vi "oa_Attach Pulse Position Info.vi"(0 "speed profile signal input":waveform(dbl)={"t0"=timestamp(0 s since 1904-01-01), "dt"=0.0, "Y"=[]}, 5 "pulse/revolution (1)":i32, 7 "Rotation direction":u16(ring) caption="rotation direction  (CCW)" items=["CCW", "CW"], 9 "speed profile input":T1 {"speed [RPM]" format="%.2f"; "time [s]" format="%.2f"}, 11 "error in (no error)":errorcluster) -> (4 "speed profile":waveform(dbl), 15 "error out":errorcluster)   [LabVIEW 2017, in "SoundVib_TachProcess.lvlib"]
uses:
  <vilib>/addons/Sound and Vibration/Order Analysis/Tach Process/SoundVib_TachProcess.lvlib
  <vilib>/addons/Sound and Vibration/Order Analysis/Tach Process/SubVIs/speed profile.ctl
panel:
  in  "Waveform":waveform(dbl)={"t0"=timestamp(0 s since 1904-01-01), "dt"=0.0, "Y"=[], "attributes"=variant("NI_OA_Pulse_Per_Rev"=variant(i32 1), "NI_OA_Rotation_Direction"=variant(u16 0), "NI_OA_Speed_Profile"=variant(cluster{"time [s]":dbl[], "speed [RPM]":dbl[]} {"time [s]"=[], "speed [RPM]"=[]}))}
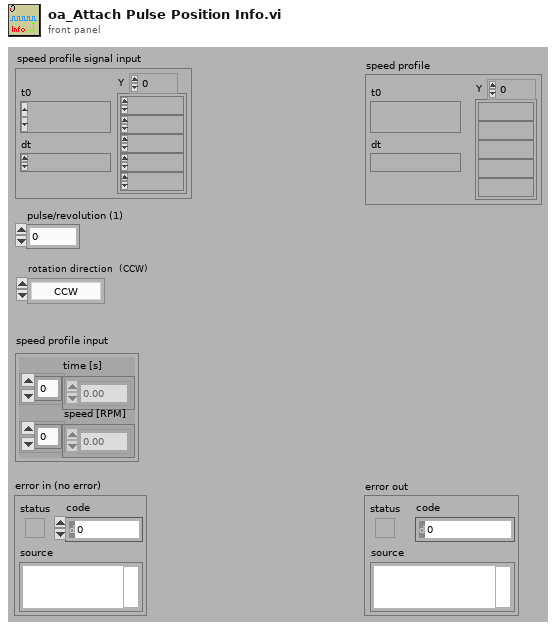
[diagram p1: front panel]
types:
  T1 = typedef "SoundVib_TachProcess.lvlib/speed profile.ctl" = cluster{"time [s]":dbl[], "speed [RPM]":dbl[]}
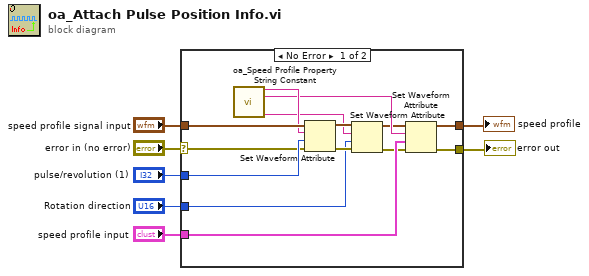
[diagram p0: block diagram]
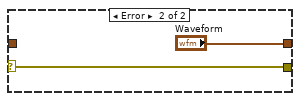
[diagram p2: hidden frame]
diagram:
  n1 = case shown="No Error" "error in (no error)" {
    selector: "error in (no error)" -> [w16 w23]
    tunnel: "speed profile signal input" -> [w21 _]
    tunnel: "pulse/revolution (1)" -> [w20 _]
    tunnel: [w19 "Waveform"] -> w5
    tunnel: [w18 w23] -> w4
    tunnel: "speed profile input" -> [w17 _]
    tunnel: "Rotation direction" -> [w8 _]
    frame No Error {
      n2 = call <vilib>:"oa_Speed Profile Property String Constant.vi"() -> ("pulse/rev"=w15:string, "speed profile"=w14:string, "rotation direction"=w9:string)  [unwired: 12 in, 1 out]
      n3 = Set Waveform Attribute(4:w16, 5:w20, 6:w15, 7:w21) -> (0:w12:errorcluster, 3:w11:waveform(dbl))  [unwired: 1 out]
      n4 = Set Waveform Attribute(4:w12, 5:w8, 6:w9, 7:w11) -> (0:w13:errorcluster, 3:w10:waveform(dbl))  [unwired: 1 out]
      n5 = Set Waveform Attribute(4:w13, 5:w17, 6:w14, 7:w10) -> (0:w18:errorcluster, 3:w19:waveform(dbl))  [unwired: 1 out]
    }
    frame Error {
    }
  }
  "error out" <- w4
  "speed profile" <- w5
